vi "Read.vi"(5 "LogSuspend":bool, 8 "error in":errorcluster, 10 "Request Number of Message":i32=1, 11 "UdsHandleIn":T2={"LogPath"=path "", "LogEnabled"=FALSE, "isOpen"=FALSE, "LogContent"="", "Adapter"="CAN0", "MCanHandle"={"MCanAdapter"=refnum}, "TransmittId"=0, "ReceiveId"=0}) -> (0 "error out":errorcluster, 2 "Messages":T1[](array[typedef]), 3 "UdsHandleOut":T2={"LogPath"=path "", "LogEnabled"=FALSE, "isOpen"=FALSE, "LogContent"="", "Adapter"="CAN0", "MCanHandle"={"MCanAdapter"=refnum}, "TransmittId"=0, "ReceiveId"=0})   [LabVIEW 2011, in "Konvolucio MUDS150628.lvlib"]
uses:
  <instrlib>/Konvolucio MUDS150628/Konvolucio MUDS150628.lvlib
  <instrlib>/Konvolucio MUDS150628/Types/UdsHandleType.ctl
  <instrlib>/Konvolucio MCAN120803/Types/MCanHandleType.ctl
  C:/Program Files/National Instruments/LabVIEW 2011/instr.lib/Konvolucio MCAN120803/Private/Konvolucio.MCAN120803.dll
  Konvolucio MCAN120803/Private/Konvolucio.MCAN120803.dll
  <instrlib>/Konvolucio MCAN120803/Types/MessageType.ctl
  <instrlib>/Konvolucio MUDS150628/Private/UdsLogCanRxMessage.vi
  <instrlib>/Konvolucio MCAN120803/Konvolucio MCAN120803.lvlib
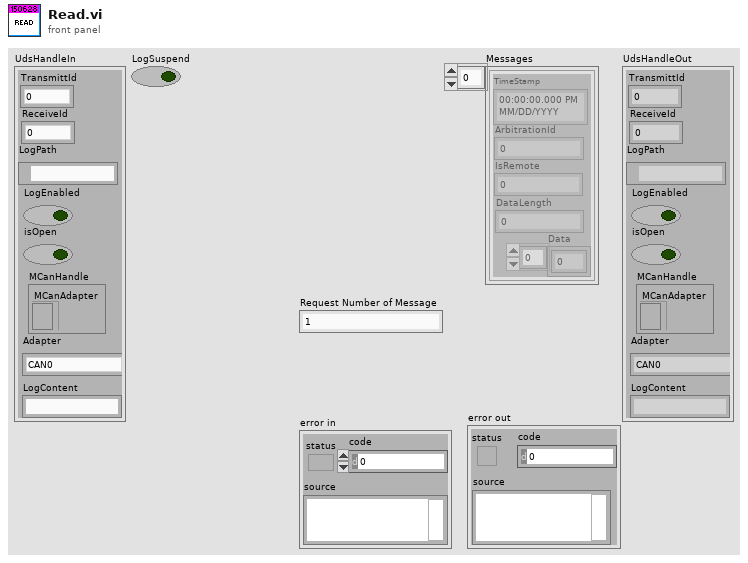
[diagram p1: front panel]
types:
  T1 = typedef "Konvolucio MCAN120803.lvlib/MessageType.ctl" = cluster{"TimeStamp":timestamp, "ArbitrationId":u32, "IsRemote":u8, "DataLength":u8, "Data":u8[]}
  T2 = typedef "Konvolucio MUDS150628.lvlib/UdsHandleType.ctl" = cluster{"LogPath":path, "LogEnabled":bool, "isOpen":bool, "LogContent":string, "Adapter":string, "MCanHandle":T3, "TransmittId":u32, "ReceiveId":u32}
  T3 = typedef "Konvolucio MCAN120803.lvlib/MCanHandleType.ctl" = cluster{"MCanAdapter":refnum<k24>}
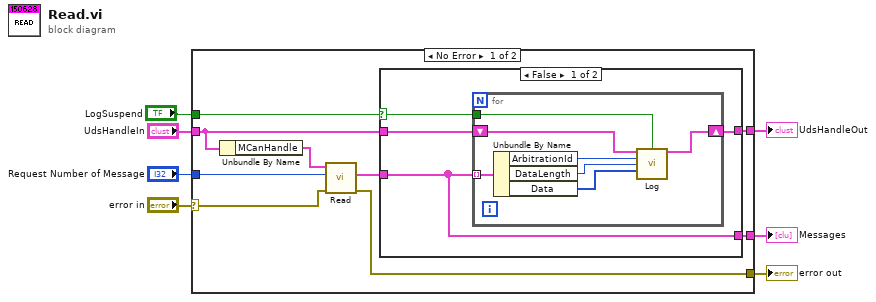
[diagram p0: block diagram]
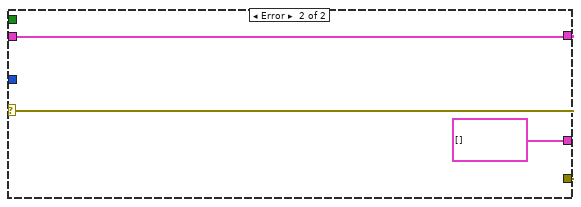
[diagram p3: hidden frame]
diagram:
  n1 = case shown="No Error" "error in" {
    selector: "error in" -> [w10 w30]
    tunnel: "UdsHandleIn" -> [w8 w32]
    tunnel: "Request Number of Message" -> [w15 _]
    tunnel: [w13 w32] -> w5
    tunnel: "LogSuspend" -> [w12 _]
    tunnel: [w11 T1[] [] ("Messages")] -> w3
    tunnel: [w9 w30] -> w1
    frame No Error {
      n2 = Unbundle By Name(w8) -> ("MCanHandle"=w16:T3)
      n3 = call <instrlib>:"Read.vi"("error in"=w10, "Request Number of Message"=w15, "MCanHandleIn"=w16) -> ("error out"=w9:errorcluster, "Messages"=w14:T1[])  [unwired: 6 in, 1 out]
      n4 = case shown="False" w12 {
        selector: w12 -> [w17 _]
        tunnel: [w20 w28] -> w13
        tunnel: w14 -> [w19 w29]
        tunnel: [w19 w29] -> w11
        tunnel: w8 -> [w18 w28]
        frame False {
          n5 = for {
            tunnel: w19 -> [w27] mode=indexing
            shift-right: [w22] -> w20
            shift-left: w18 -> [w23]
            tunnel: w17 -> [w21]
            n6 = Unbundle By Name(w27) -> ("ArbitrationId"=w26:u32, "DataLength"=w25:u8, "Data"=w24:u8[])
            n7 = call-poly <instrlib>:"Log.vi"("UdsHandleIn"=w23, "LogSuspend"=w21, "Id"=w26, "DataLength"=w25, "Data"=w24) -> ("UdsHandleOut"=w22:T2)  [unwired: 9 in, 1 out]
          }
        }
        frame True {
        }
      }
    }
    frame Error {
    }
  }
  "error out" <- w1
  "UdsHandleOut" <- w5
  "Messages" <- w3
